vi "peg-in-hole Test.vi"() -> ()   [LabVIEW 2013]
uses:
  ROS/Code/SubVIs/BaxterSide.ctl
  Arm Globals.vi
  ROS/Code/Console/Servers/ServerSubs/(nist) Arm Globals.vi
panel:
  in  "Load Start":bool
  in  "Joint Pose":dbl[](array[numeric])=[36.057128865048725, -54.909667906006554, 15.051269514051416, 106.23779284735562, -16.325683575095187, 38.45214839356202, 18.808593728508047]
  in  "Peg Positions":i32[](array[numeric])
  out "Loops Remaining":i32=1
  out "Peg":i32=1
  out "Times":dbl[](array[numeric])=[15.75, 15.9, 16.0, 15.85, 15.85, 15.4, 15.65, 15.8, 15.75, 15.75, 15.9, 16.0, 15.75, 15.5, 15.700000000000001, 15.6, 15.85, 15.8, 15.6, 15.8, 15.5, 15.5, 15.75, 15.55, 15.450000000000001, 15.8, 15.5, 15.450000000000001, 15.6, 15.4, 15.3, 25.35, 15.6, 15.65, 15.700000000000001, 25.0, 15.65, 15.450000000000001, 15.8, 15.8, 15.549, 16.0, 15.6, 15.5, 15.6, 15.55, 24.75, 15.55, 16.4, 16.049, 16.05, 16.05, 16.3, 15.85, 15.55, 15.65, 15.75, 16.35, 25.85, 25.400000000000002, 16.2, 15.9, 16.2, 15.950000000000001, 15.950000000000001, 15.35, 15.75, 53.0, 15.450000000000001, 15.700000000000001, 15.450000000000001, 35.5, 15.25, 15.501, 33.3, 25.2, 15.6, 25.400000000000002, 15.55, 15.5, 16.0, 15.700000000000001, 15.65, 32.7, 15.4, 15.55, 15.65, 15.65, 15.6, 15.55, 15.85, 15.75, 15.9, 15.65, 15.65, 15.450000000000001, 15.700000000000001, 15.6, 16.0, 15.4, 15.8, 15.55, 15.700000000000001, 24.05, 15.55, 15.85, 15.9, 15.6, 15.9, 15.8, 15.700000000000001, 15.6, 15.450000000000001, 24.0, 15.35, 15.700000000000001, 15.65, 15.85, 15.450000000000001, 15.700000000000001, 15.85, 15.55, 16.1, 15.6, 15.700000000000001, 15.499, 15.8, 15.55, 15.950000000000001, 15.450000000000001, 15.35, 16.0, 15.6, 15.6, 15.700000000000001, 15.6, 15.75, 15.75, 15.450000000000001, 15.35]
  out "Status":string="Test.4"
  in  "Stop":bool
  out "error out":errorcluster
  # "1\n2\n3\n4\n5\n6\n7"
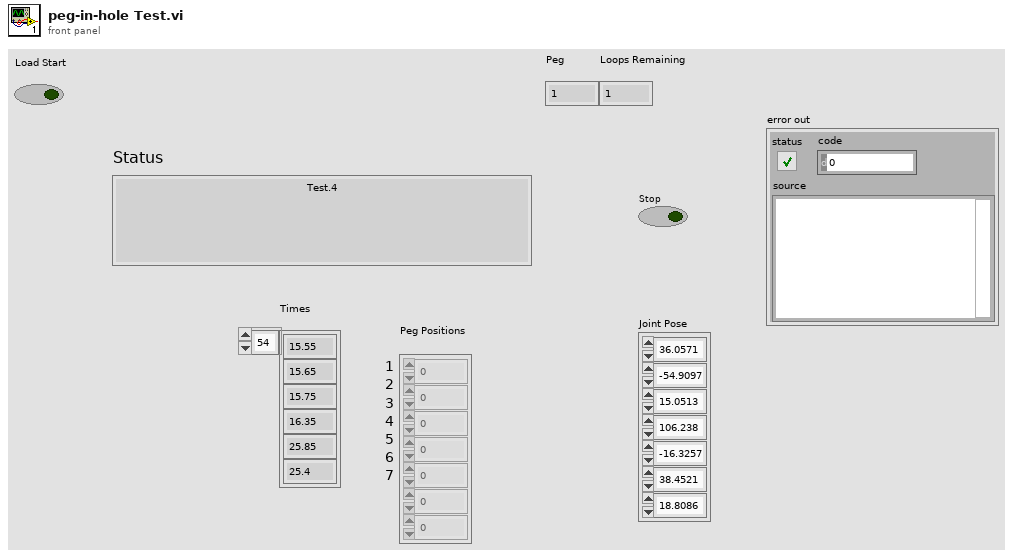
[diagram p1: front panel]
types:
  T1 = cluster{"X":dbl, "Y":dbl, "Z":dbl, "O":dbl, "A":dbl, "T":dbl}
  T2 = typedef "BaxterSide.ctl" = enum16{"left", "right"}
  T3 = cluster{"X":dbl, "Y":dbl, "Z":dbl, "O":dbl, "A":dbl, "T":dbl}[]
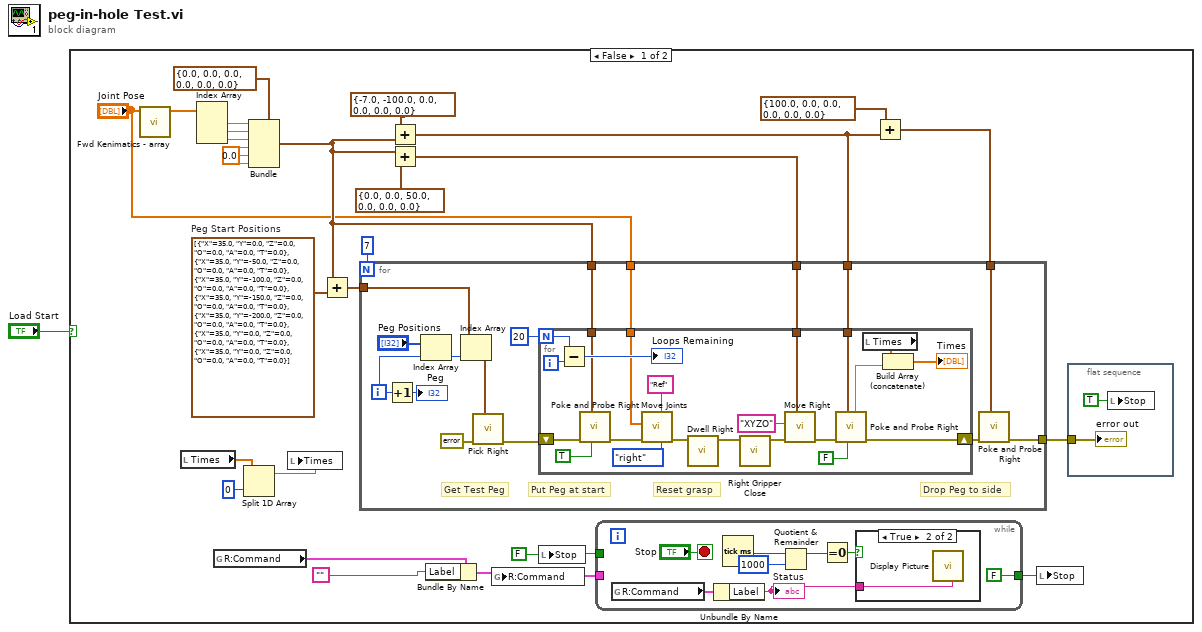
[diagram p0: block diagram]
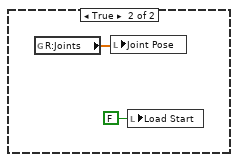
[diagram p3: hidden frame]
diagram:
  n1 = case shown="False" "Load Start" {
    frame False {
      w8 = FALSE ("Stop")
      w13 = 0.0 ("A")
      w20 = T3 [{"X"=35.0, "Y"=0.0, "Z"=0.0, "O"=0.0, "A"=0.0, "T"=0.0}, {"X"=35.0, "Y"=-50.0, "Z"=0.0, "O"=0.0, "A"=0.0, "T"=0.0}, {"X"=35.0, "Y"=-100.0, "Z"=0.0, "O"=0.0, "A"=0.0, "T"=0.0}, {"X"=35.0, "Y"=-150.0, "Z"=0.0, "O"=0.0, "A"=0.0, "T"=0.0}, {"X"=35.0, "Y"=-200.0, "Z"=0.0, "O"=0.0, "A"=0.0, "T"=0.0}, {"X"=35.0, "Y"=0.0, "Z"=0.0, "O"=0.0, "A"=0.0, "T"=0.0}, {"X"=35.0, "Y"=0.0, "Z"=0.0, "O"=0.0, "A"=0.0, "T"=0.0}]  # Peg Start Positions
      n2 = call "Fwd Kenimatics - array.vi"("Joints"="Joint Pose") -> ("Position"=w18:dbl[])  [unwired: 9 in, 1 out]
      n3 = local read "Times"() -> (w26:dbl[])
      n4 = Index Array(array=w18) -> (element #1=w15:dbl, element #2=w17:dbl, element #3=w14:dbl)  [unwired: 3 in]
      n5 = global read "Arm Globals.vi" "R:Command"() -> (w4:cluster{"Label":string, "Angles":dbl[]})
      n6 = Split 1D Array(array=w26, index=0) -> (first subarray=w24:dbl[])  [unwired: 1 out]
      n7 = Bundle(cluster=T1 {"X"=0.0, "Y"=0.0, "Z"=0.0, "O"=0.0, "A"=0.0, "T"=0.0} ("Left Hole"), "X"=w15, "Y"=w17, "Z"=w14, "O"=w13, "A"=w13, "T"=w13) -> (w3:T1)
      n8 = local write "Times"(w24) -> ()
      n9 = Add(x=w3, y=w20) -> (x+y=w23:T3)
      n10 = Add(x=T1 {"X"=-7.0, "Y"=-100.0, "Z"=0.0, "O"=0.0, "A"=0.0, "T"=0.0}, y=w3) -> (x+y=w9:T1)
      n11 = Add(x=w3, y=T1 {"X"=0.0, "Y"=0.0, "Z"=50.0, "O"=0.0, "A"=0.0, "T"=0.0} ("x")) -> (x+y=w12:T1)
      n12 = Bundle By Name(cluster=w4, "Label"="") -> (w6:cluster{"Label":string, "Angles":dbl[]})
      n13 = global write "Arm Globals.vi" "R:Command"(w6) -> ()
      n14 = local write "Stop"(w8) -> ()
      n15 = while {
        tunnel: w6 -> [_]
        tunnel: [FALSE] -> w7
        tunnel: w8 -> [_]
        stop <- "Stop" stop-if-true
        n16 = global read "Arm Globals.vi" "R:Command"() -> (w35:cluster{"Label":string, "Angles":dbl[]})
        n17 = Unbundle By Name(w35) -> ("Label"=w28:string)
        "Status" <- w28
        n18 = Tick Count (ms)() -> (millisecond timer value=w32:u32)
        n19 = Quotient & Remainder(x=w32, y=u32 1000) -> (x-y*floor(x/y)=w30:u32)  [unwired: 1 out]
        n20 = Equal To 0?(x=w30) -> (x = 0?=w29:bool)
        n21 = case shown="True" w29 {
          tunnel: w28 -> [_ w36]
          frame False {
          }
          frame True {
            n22 = call "Display Picture.vi"("Comment"=w36) -> ()  [unwired: 10 in, 1 out]
          }
        }
      }
      n23 = Add(x=T1 {"X"=100.0, "Y"=0.0, "Z"=0.0, "O"=0.0, "A"=0.0, "T"=0.0}, y=w9) -> (x+y=w21:T1)
      n24 = for {
        N: 7 -> [_]
        tunnel: [w48] -> w27
        tunnel: w23 -> [w47]
        tunnel: w9 -> [w49]
        tunnel: w21 -> [w50]
        tunnel: w12 -> [w40]
        tunnel: w3 -> [w39]
        tunnel: "Joint Pose" -> [w38]
        i -> [w44]
        # "Reset grasp"
        # "Put Peg at start"
        # "Drop Peg to side"
        # "Get Test Peg"
        n25 = Increment(x=w44) -> (x+1=→"Peg":i32)
        n26 = Index Array(array="Peg Positions", index=w44) -> (element=w43:i32)
        n27 = Index Array(array=w47, index=w43) -> (element=w46:T1)
        n28 = call "Pick Right.vi"("Pick"=w46, "error in"=errorcluster {"status"=FALSE, "code"=0, "source"=""}) -> ("error out"=w42:errorcluster)  [unwired: 8 in, 1 out]
        n29 = for {
          N: 20 -> [w73]
          shift-right: [w60] -> w41
          shift-left: w42 -> [w67]
          tunnel: w49 -> [w70]
          tunnel: w40 -> [w59]
          tunnel: w38 -> [w58]
          tunnel: w39 -> [w57]
          i -> [w72]
          n30 = Subtract(x=w73, y=w72) -> (x-y=→"Loops Remaining":i32)
          n31 = call "Poke and Probe Right.vi"("Release Part"=TRUE, "Goal"=w57, "error in"=w67) -> ("error out"=w66:errorcluster)  [unwired: 6 in, 2 out]
          n32 = call "Move Joints.vi"("Side"=BaxterSide."right", "Label"="Ref", "error in"=w66, "Goal"=w58) -> ("error out"=w65:errorcluster)  [unwired: 6 in, 1 out]
          n33 = call "Dwell Right.vi"("error in"=w65) -> ("error out"=w54:errorcluster)  [unwired: 10 in]
          n34 = call "Right Gripper Close.vi"("error in"=w54) -> ("error out"=w64:errorcluster)  [unwired: 9 in, 1 out]
          n35 = call "Move Right.vi"("Goal"=w59, "error in"=w64, "Mask"="XYZO") -> ("error out"=w62:errorcluster)  [unwired: 4 in, 4 out]
          n36 = call "Poke and Probe Right.vi"("Release Part"=FALSE, "Goal"=w70, "error in"=w62) -> ("error out"=w60:errorcluster, "time"=w53:dbl)  [unwired: 6 in, 1 out]
          n37 = local read "Times"() -> (w63:dbl[])
          n38 = Build Array (concatenate)(w63, w53) -> (→"Times":dbl[])
        }
        n39 = call "Poke and Probe Right.vi"("Goal"=w50, "error in"=w41) -> ("error out"=w48:errorcluster)  [unwired: 7 in, 2 out]
      }
      n40 = local write "Stop"(w7) -> ()
      n41 = flat-sequence {
        tunnel: w27 -> [w76]
        frame #0 {
          n42 = local write "Stop"(TRUE ("Stop")) -> ()
          "error out" <- w76
        }
      }
    }
    frame True {
      n43 = global read "(nist) Arm Globals.vi" "R:Joints"() -> (w78:dbl[])
      n44 = local write "Joint Pose"(w78) -> ()
      n45 = local write "Load Start"(FALSE ("Load Start")) -> ()
    }
  }
